vi "Lang Set Desc Frame Basic.vi"(8 "error in (no error)":errorcluster, 9 "Frame Skill":T1, 10 "Frame Basic":T3, 11 "LF2R IDE in":refnum<class "Main Panel.lvclass">) -> (0 "error out":errorcluster, 3 "LF2R IDE out":refnum<class "Main Panel.lvclass">)   [LabVIEW 2018, in "Framework.lvlib" / "Framework.lvclass"]
uses:
  Framework/Framework/Framework.lvclass
  Main Panel.lvclass
  D:/project/hobby/LabVIEW/LF2R/LabVIEW/Source/Actor/Framework/Framework/Framework.lvclass
  C:/Program Files (x86)/National Instruments/LabVIEW 2018/vi.lib/MGI/Panel Manager/Panel Actor/Panel Actor/Panel Actor.lvclass
  C:/Program Files (x86)/National Instruments/LabVIEW 2018/vi.lib/MGI/Monitored Actor/Monitored Actor/Monitored Actor/Monitored Actor.lvclass
  C:/Program Files (x86)/National Instruments/LabVIEW 2018/vi.lib/ActorFramework/Actor/Actor.lvclass
  Const Lang Property.ctl
  Const UI Desc Frame Basic.ctl
  Const UI Desc Frame Skill.ctl
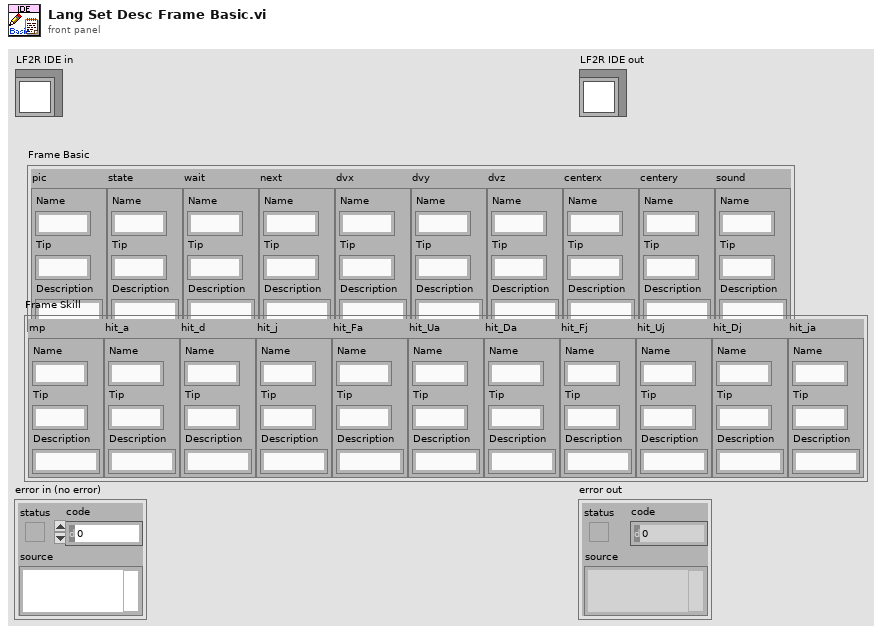
[diagram p1: front panel]
types:
  T1 = typedef "Framework.lvlib/Framework.lvclass/Const UI Desc Frame Skill.ctl" = cluster{"mp":T2, "hit_a":T2, "hit_d":T2, "hit_j":T2, "hit_Fa":T2, "hit_Ua":T2, "hit_Da":T2, "hit_Fj":T2, "hit_Uj":T2, "hit_Dj":T2, "hit_ja":T2}
  T2 = typedef "Framework.lvlib/Framework.lvclass/Const Lang Property.ctl" = cluster{"Name":string, "Tip":string, "Description":string}
  T3 = typedef "Framework.lvlib/Framework.lvclass/Const UI Desc Frame Basic.ctl" = cluster{"pic":T2, "state":T2, "wait":T2, "next":T2, "dvx":T2, "dvy":T2, "dvz":T2, "centerx":T2, "centery":T2, "sound":T2}
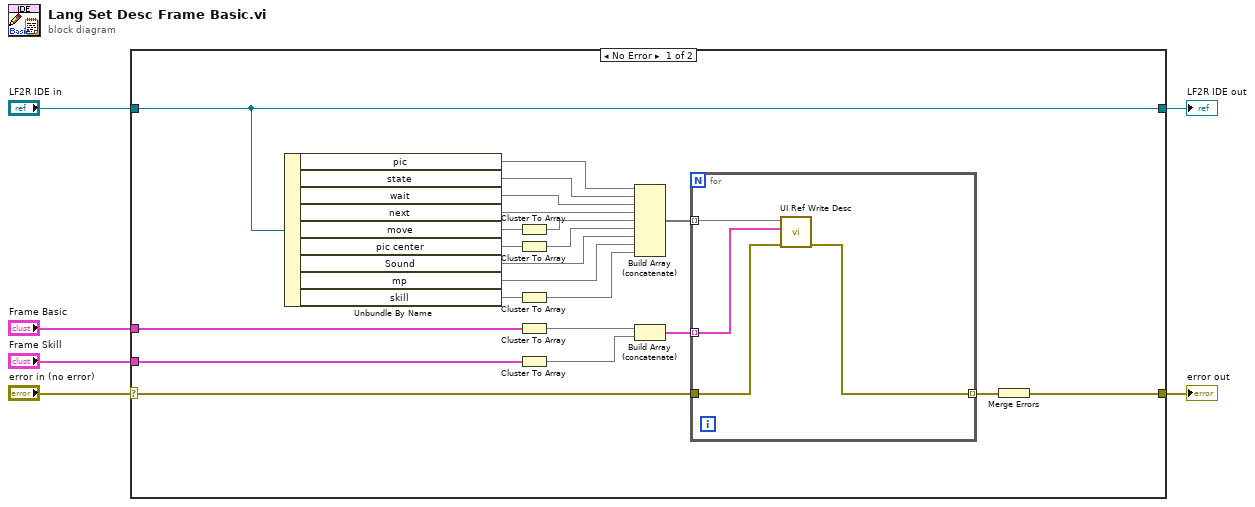
[diagram p0: block diagram]
diagram:
  n1 = case shown="No Error" "error in (no error)" {
    selector: "error in (no error)" -> [w14 w34]
    tunnel: [w12 w34] -> w5
    tunnel: [w28 w33] -> w3
    tunnel: "LF2R IDE in" -> [w28 w33]
    tunnel: "Frame Basic" -> [w19 _]
    tunnel: "Frame Skill" -> [w18 _]
    frame No Error {
      n2 = Unbundle By Name(w28) -> ("pic"=w10, "state"=w9, "wait"=w8, "next"=w7, "move"=w27, "pic center"=w25, "Sound"=w11, "mp"=w22, "skill"=w26)
      n3 = Cluster To Array(cluster=w27) -> (array=w24:void[])
      n4 = Cluster To Array(cluster=w25) -> (array=w23:void[])
      n5 = Cluster To Array(cluster=w26) -> (array=w21:void[])
      n6 = Cluster To Array(cluster=w19) -> (array=w17:T2[])
      n7 = Cluster To Array(cluster=w18) -> (array=w16:T2[])
      n8 = Build Array (concatenate)(w10, w9, w8, w7, w24, w23, w11, w22, w21) -> (w20:void[])
      n9 = Build Array (concatenate)(w17, w16) -> (w15:T2[])
      n10 = for {
        tunnel: w20 -> [w32] mode=indexing
        tunnel: w15 -> [w31] mode=indexing
        tunnel: w14 -> [w30]
        tunnel: [w29] -> w13 mode=indexing
        n11 = call "UI Ref Write Desc.vi"("error in (no error)"=w30, "UI Property"=w31, "UI Ref"=w32) -> ("error out"=w29:errorcluster)  [unwired: 8 in]
      }
      n12 = Merge Errors(w13) -> (w12:errorcluster)
    }
    frame Error {
    }
  }
  "error out" <- w5
  "LF2R IDE out" <- w3
